vi "Get Train Rate (No Objects).vi"(10 "going up?":bool=TRUE, 11 "Cluster In":T4={"Field"=0.0, "Rate"=0.0, "Status"={"Sweeping"=FALSE, "Clamped"=FALSE, "Hold"=FALSE, "At Rest"=FALSE, "Quench"=FALSE, "Persistent Mode"=FALSE, "Switch Heater"=FALSE}, "ILM Shut Down?"=FALSE, "IO Info"={"Address"={"Com Port"=1, "ISOBUS Address"=2, "GPIB Address"=24, "Communication"=enum."ISOBUS"}, "Version"=enum."IPS"}, "IO Info (Level Meter)"={"Address"={"Com Port"=1, "ISOBUS Address"=5, "GPIB Address"=24, "Communication"=enum."ISOBUS"}, "ILM Name"="", "Display Channel"=[]}, "Training?"=FALSE, "Training Field and Speed Cluster"={"Training Field"=[0.0, 4.108, 5.78, 8.001], "Training Speed"=[0.0057, 0.0022833333333333334, 0.0011333333333333334, 0.0011333333333333334]}}) -> (2 "Rate Out":dbl[unit]=0.11666666666666667, 3 "Cluster Out":T4={"Field"=0.0, "Rate"=0.0, "Status"={"Sweeping"=FALSE, "Clamped"=FALSE, "Hold"=FALSE, "At Rest"=FALSE, "Quench"=FALSE, "Persistent Mode"=FALSE, "Switch Heater"=FALSE}, "ILM Shut Down?"=FALSE, "IO Info"={"Address"={"Com Port"=1, "ISOBUS Address"=2, "GPIB Address"=24, "Communication"=enum."ISOBUS"}, "Version"=enum."IPS"}, "IO Info (Level Meter)"={"Address"={"Com Port"=1, "ISOBUS Address"=5, "GPIB Address"=24, "Communication"=enum."ISOBUS"}, "ILM Name"="", "Display Channel"=[]}, "Training?"=FALSE, "Training Field and Speed Cluster"={"Training Field"=[0.0, 4.108, 5.78, 8.001], "Training Speed"=[0.0057, 0.0022833333333333334, 0.0011333333333333334, 0.0011333333333333334]}})   [LabVIEW 2009]
uses:
  Magnet status.ctl
  Oxford/PSSUBS.LLB/PSIO.ctl
  Oxford/BUSGEN.LLB/OxfordAddress.ctl
  Power Supply.lvclass
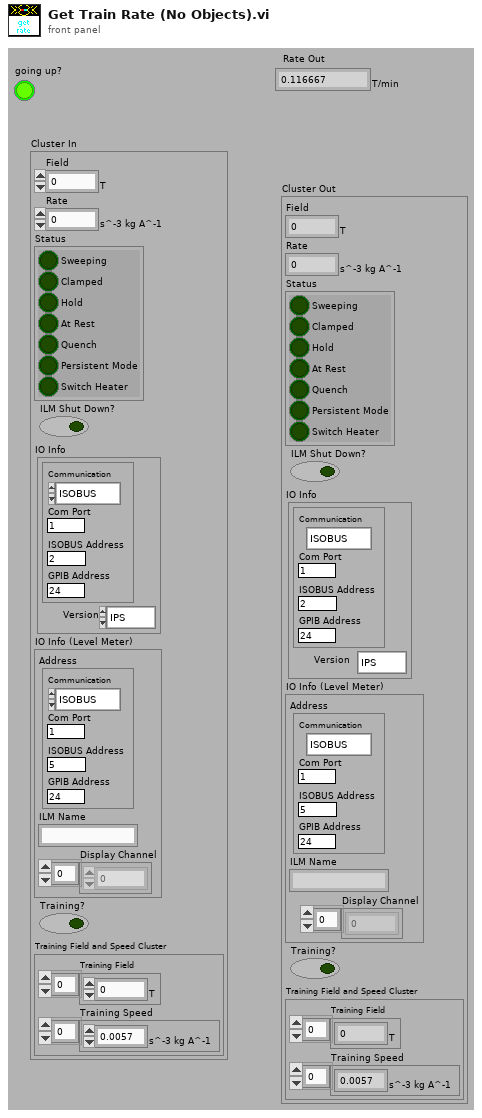
[diagram p1: front panel]
types:
  T1 = typedef "Power Supply.lvclass/Magnet status.ctl" = cluster{"Sweeping":bool, "Clamped":bool, "Hold":bool, "At Rest":bool, "Quench":bool, "Persistent Mode":bool, "Switch Heater":bool}
  T2 = typedef "PSIO.ctl" = cluster{"Address":T3, "Version":enum16{"PS", "IPS"}}
  T3 = typedef "OxfordAddress.ctl" = cluster{"Com Port":i32, "ISOBUS Address":i32, "GPIB Address":i16, "Communication":enum16{"RS232", "ISOBUS", "GPIB", "Gateway"}}
  T4 = cluster{"Field":dbl[unit], "Rate":dbl[unit], "Status":T1, "ILM Shut Down?":bool, "IO Info":T2, "IO Info (Level Meter)":cluster{"Address":T3, "ILM Name":string, "Display Channel":i32[]}, "Training?":bool, "Training Field and Speed Cluster":cluster{"Training Field":dbl[unit][], "Training Speed":dbl[unit][]}}
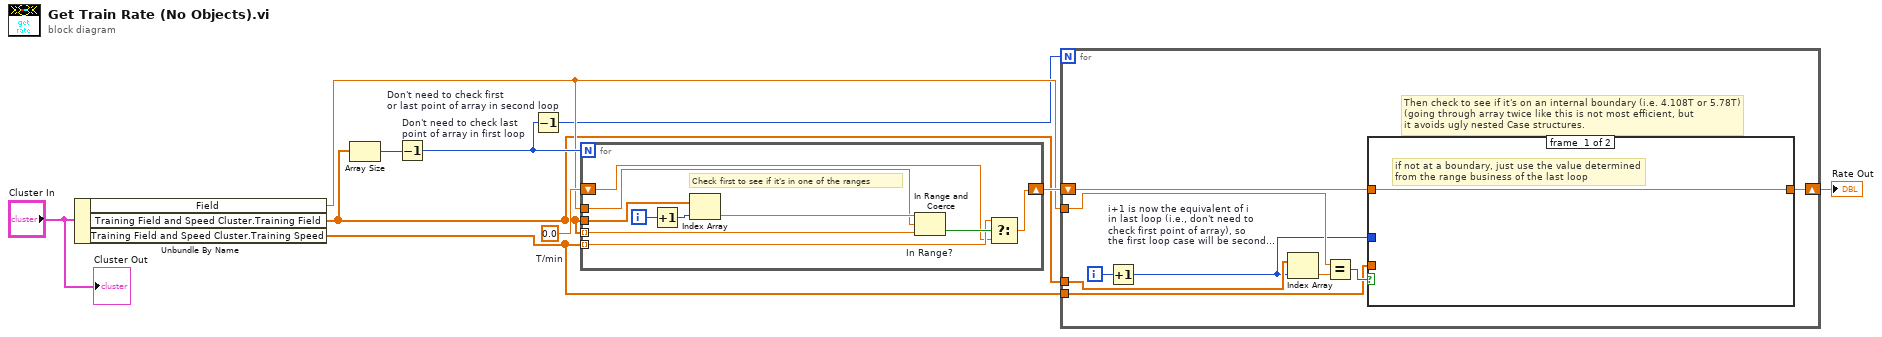
[diagram p0: block diagram]
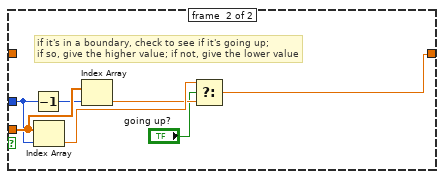
[diagram p2: hidden frame]
diagram:
  w9 = dbl[unit] 0.0  # T/min
  n1 = Unbundle By Name("Cluster In") -> ("Field"=w5:dbl[unit], "Training Field and Speed Cluster.Training Field"=w4:dbl[unit][], "Training Field and Speed Cluster.Training Speed"=w3:dbl[unit][])
  n2 = Array Size(array=w4) -> (size(s)=w10:i32)
  n3 = Decrement "Don't need to check last \npoint of array in first loop"(x=w10) -> (x-1=w6:i32)
  n4 = Decrement "Don't need to check first\nor last point of array in second loop"(x=w6) -> (x-1=w2:i32)
  n5 = for {
    N: w6 -> [_]
    tunnel: w5 -> [w17]
    tunnel: w4 -> [w16]
    tunnel: w4 -> [w15] mode=indexing
    tunnel: w3 -> [w13] mode=indexing
    shift-right: [w12] -> w8
    shift-left: w9 -> [w11]
    i -> [w18]
    # "Check first to see if it's in one of the ranges"
    n6 = Increment(x=w18) -> (x+1=w19:i32)
    n7 = Index Array(array=w16, index=w19) -> (element=w20:dbl[unit])
    n8 = In Range and Coerce "In Range?"(upper limit=w20, x=w17, lower limit=w15) -> (In Range?=w14:bool)  [unwired: 1 out]
    n9 = Select(t=w13, s=w14, f=w11) -> (s? t:f=w12:dbl[unit])
  }
  n10 = for {
    N: w2 -> [_]
    tunnel: w5 -> [w26]
    tunnel: w4 -> [w24]
    tunnel: w3 -> [w22]
    shift-right: [w28] -> w7
    shift-left: w8 -> [w27]
    i -> [w29]
    # "Then check to see if it's on an internal boundary (i.e. 4.108T or 5.78T)\n(going through array twice like this is not most efficient, but\nit avoids ugly nested Case structures."
    n11 = Increment "i+1 is now the equivalent of i\nin last loop (i.e., don't need to \ncheck first point of array), so \nthe first loop case will be second\npoint"(x=w29) -> (x+1=w21:i32)
    n12 = Index Array(array=w24, index=w21) -> (element=w23:dbl[unit])
    n13 = Equal?(x=w26, y=w23) -> (x = y?=w25:bool)
    n14 = case shown="True" w25 {
      tunnel: [w30 w37] -> w28
      tunnel: w27 -> [w30 _]
      tunnel: w22 -> [_ w36]
      tunnel: w21 -> [_ w34]
      frame #0 {
        # "if not at a boundary, just use the value determined \nfrom the range business of the last loop"
      }
      frame #1 {
        # "if it's in a boundary, check to see if it's going up; \nif so, give the higher value; if not, give the lower value"
        n15 = Decrement(x=w34) -> (x-1=w35:i32)
        n16 = Index Array(array=w36, index=w34) -> (element=w33:dbl[unit])
        n17 = Index Array(array=w36, index=w35) -> (element=w32:dbl[unit])
        n18 = Select(t=w33, s="going up?", f=w32) -> (s? t:f=w37:dbl[unit])
      }
    }
  }
  "Rate Out" <- w7
  "Cluster Out" <- "Cluster In"
